vi "Sandbox.vi"() -> ()   [LabVIEW 2019, in "FPGA API.lvclass"]
uses:
  FPGA API.lvclass
  FPGA/TypeDef/DO index.ctl
  <vilib>/ptbypt/NI_PtbyPt.lvlib
panel:
  out "Ds":bool[](array[boolean])
  in  "#DO":T1 items=["DO 0 [KP1 [DO 0]]", "DO 1 [ON KP2 [DO 1]]", "DO 2 [ON KP3 [DO 2]]", "DO 3 [WATER Y18.1 [DO3]]", "DO 4 [WATER Y18.2 [DO4]]", "DO 5 [KP6 Y29.1 33.7]", "DO 6 [KP7 Y29.2 33.8]", "DO 7 [KP8 Y29.3 33.9]", "DO 8 [KP9 Y29.4  33.12]", "DO 9 [KP10 Y29.5 33.1]", "DO 10 [KP11 Y29.6 33.2]", "DO 11 [KP12 Y29.7  33.13]", "DO 12 [KP13 Y29.8  33.11]", "DO 13 [KP14 Y29.9 33.10]", "DO 14 [KP15 Y29.10  33.6]", "DO 15 [KP16 Y29.11  33.5]", "DO 16 [KP17 Y29.12  33.4]", "DO 17 [KP18 Y29.13 33.3]", "DO 18 [AIR KP19]", "DO 19 [STEP DRIVE EN KP20]", "DO 20 [KP21 Y44.1 OPEN]", "DO 21 [ KP22 Y44.1 CLOSE]", "DO 22 [ KP23 Y44.2 OPEN]", "DO 23", "DO 24 [STEP DRIVE 1]", "DO 25 [STEP DRIVE 2]"]
  out "Numeric":i32
  out "filter %":dbl
  out "avr %":dbl
  out "Raw %":dbl
  out "Waveform Chart":dbl[][](graph)
  out "DIs":bool[](array[boolean])
  out "dt(tiks) DI loop":u32
  out "dt(tiks) DO loop":u32
  out "dt(tiks) AI loop":u32
  out "error out":errorcluster
  in  "set":bool
  in  "Time uSec":u32
  in  "value":bool
  in  "stop":bool
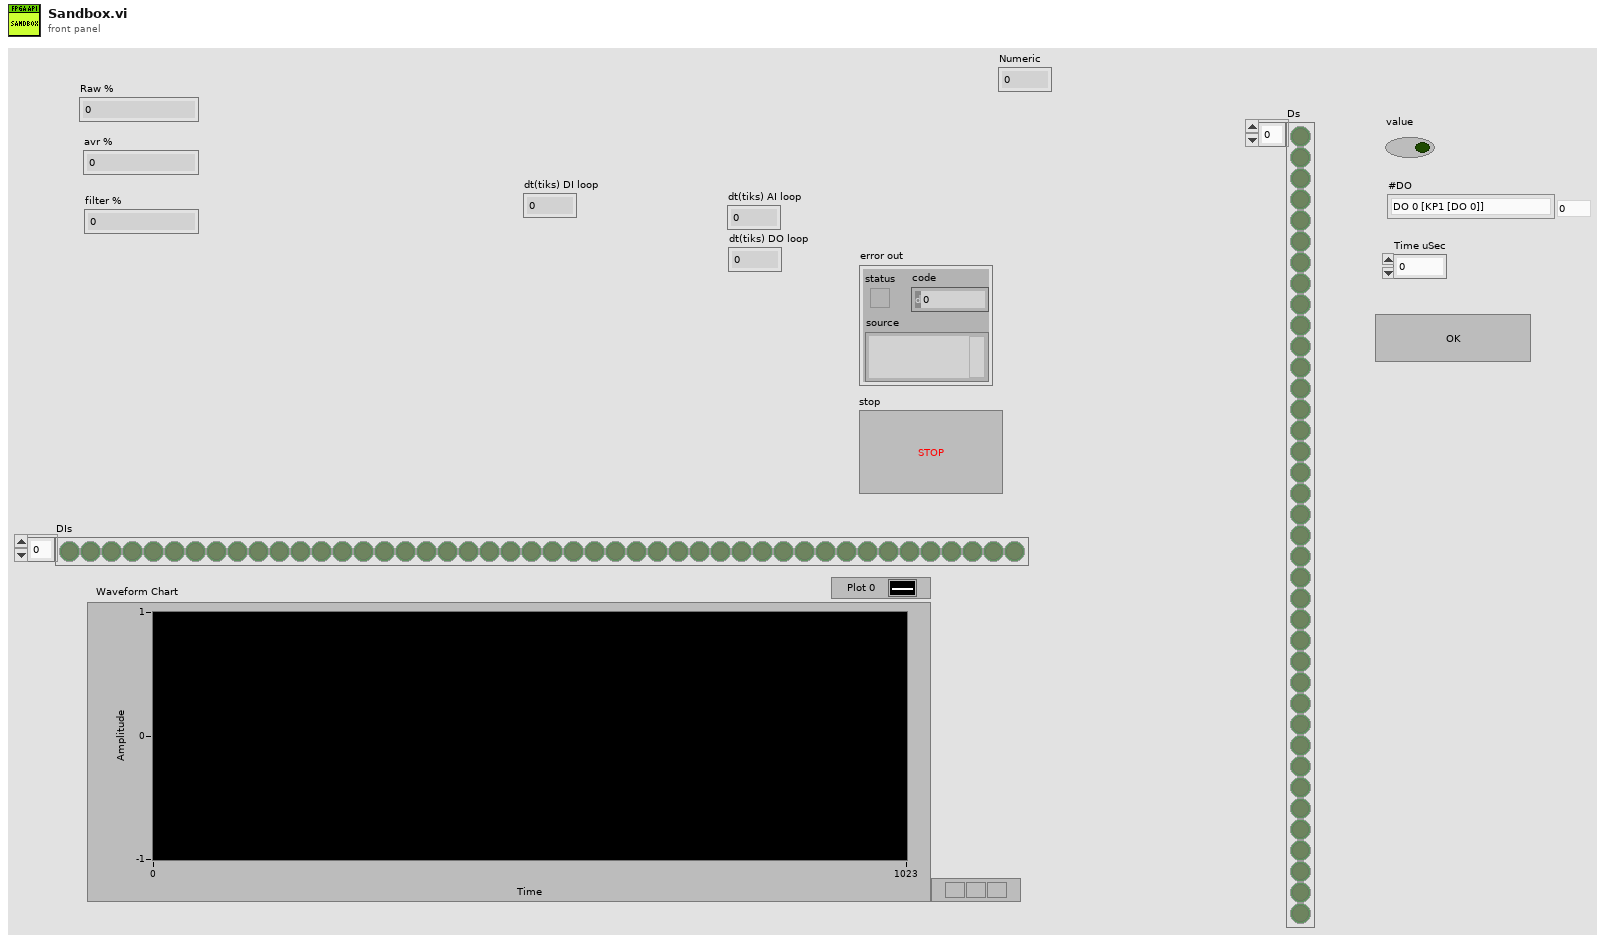
[diagram p1: front panel]
types:
  T1 = typedef "DO index.ctl" = u8
  T2 = cluster{"AI_0 L5.1":fxp<+/-,21,-4>, "AI_1 T4.1":fxp<+/-,21,-4>, "AI_2 L5.2":fxp<+/-,21,-4>, "AI_3 T4.2":fxp<+/-,21,-4>, "AI_4 V":fxp<+/-,21,-4>, "AI_5 P38.1":fxp<+/-,21,-4>, "AI_6 P38.2":fxp<+/-,21,-4>, "AI_7 P38.3":fxp<+/-,21,-4>, "AI_8 P41.1":fxp<+/-,21,-4>, "AI_9 P41.2":fxp<+/-,21,-4>, "AI_10 P41.3":fxp<+/-,21,-4>, "AI_11":fxp<+/-,21,-4>, "AI_12":fxp<+/-,21,-4>, "AI_13":fxp<+/-,21,-4>, "AI_14":fxp<+/-,21,-4>, "AI_15":fxp<+/-,21,-4>}
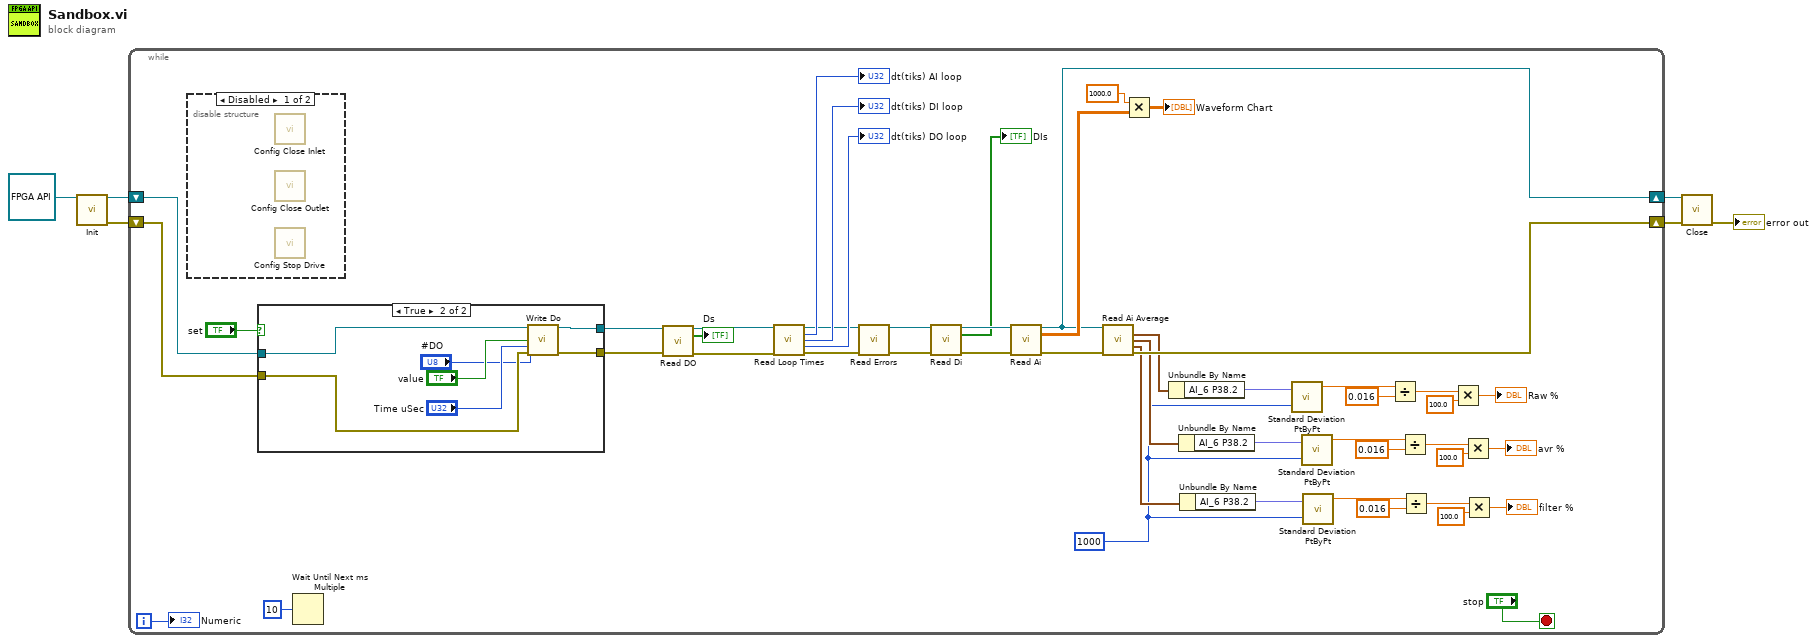
[diagram p0: block diagram]
diagram:
  n1 = call "Init.vi"("FPGA API in"=refnum<class "FPGA API.lvclass"> refnum) -> ("FPGA API out"=w5:refnum<class "FPGA API.lvclass">, "error out"=w4:errorcluster)  [unwired: 13 in]
  n2 = while {
    shift-right: [w38] -> w3
    shift-left: w5 -> [w42]
    shift-right: [w36] -> w2
    shift-left: w4 -> [w41]
    i -> [w13]
    stop <- "stop" stop-if-true
    w14 = 1000 ("sample length")
    n3 = disable-structure shown="Disabled" {
      frame Disabled {
        n4 = call "Config Close Inlet.vi"() -> ()  [unwired: 14 in, 2 out]
        n5 = call "Config Close Outlet.vi"() -> ()  [unwired: 14 in, 2 out]
        n6 = call "Config Stop Drive.vi"() -> ()  [unwired: 14 in, 2 out]
      }
      frame Enabled {
      }
    }
    n7 = case shown="True" "set" {
      tunnel: [w57 w64] -> w11
      tunnel: [w56 w63] -> w9
      tunnel: w42 -> [w57 w59]
      tunnel: w41 -> [w56 w62]
      frame False {
      }
      frame True {
        n8 = call "Write Do.vi"("FPGA API in"=w59, "#DO"="#DO", "value"="value", "Time uSec"="Time uSec", "error in (no error)"=w62) -> ("FPGA API out"=w64:refnum<class "FPGA API.lvclass">, "error out"=w63:errorcluster)  [unwired: 9 in]
      }
    }
    n9 = Wait Until Next ms Multiple(millisecond multiple=u32 10) -> ()  [unwired: 1 out]
    n10 = call "Read DO.vi"("FPGA API in"=w11, "error in (no error)"=w9) -> ("FPGA API out"=w10:refnum<class "FPGA API.lvclass">, "Ds"=→"Ds":bool[], "error out"=w8:errorcluster)  [unwired: 11 in]
    n11 = call "Read Loop Times.vi"("FPGA API in"=w10, "error in (no error)"=w8) -> ("FPGA API out"=w48:refnum<class "FPGA API.lvclass">, "dt(tiks) AI loop"=→"dt(tiks) AI loop":u32, "dt(tiks) DI loop"=→"dt(tiks) DI loop":u32, "dt(tiks) DO loop"=→"dt(tiks) DO loop":u32, "error out"=w49:errorcluster)  [unwired: 8 in, 1 out]
    n12 = call "Read Errors.vi"("FPGA API in"=w48, "error in (no error)"=w49) -> ("FPGA API out"=w47:refnum<class "FPGA API.lvclass">, "error out"=w46:errorcluster)  [unwired: 8 in, 4 out]
    n13 = call "Read Di.vi"("FPGA API in"=w47, "error in (no error)"=w46) -> ("FPGA API out"=w44:refnum<class "FPGA API.lvclass">, "DIs"=→"DIs":bool[], "error out"=w45:errorcluster)  [unwired: 11 in]
    n14 = call "Read Ai.vi"("FPGA API in"=w44, "error in (no error)"=w45) -> ("FPGA API out"=w38:refnum<class "FPGA API.lvclass">, "AI Data"=w40:dbl[][], "error out"=w37:errorcluster)  [unwired: 10 in, 1 out]
    n15 = call "Read Ai Average.vi"("FPGA API in"=w38, "error in (no error)"=w37) -> ("Raw"=w35:T2, "Average 1ms"=w16:T2, "Discrete Control Filter"=w15:T2, "error out"=w36:errorcluster)  [unwired: 9 in, 1 out]
    n16 = Multiply(x=1000.0, y=w40) -> (x*y=→"Waveform Chart":dbl[][])
    n17 = Unbundle By Name(w35) -> ("AI_6 P38.2"=w34:fxp<+/-,21,-4>)
    n18 = Unbundle By Name(w16) -> ("AI_6 P38.2"=w23:fxp<+/-,21,-4>)
    n19 = Unbundle By Name(w15) -> ("AI_6 P38.2"=w22:fxp<+/-,21,-4>)
    n20 = call <vilib>:"Standard Deviation PtByPt.vi"("x"=w34, "sample length"=w14) -> ("standard deviation"=w33:dbl)  [unwired: 1 in, 2 out]
    n21 = call <vilib>:"Standard Deviation PtByPt.vi"("x"=w23, "sample length"=w14) -> ("standard deviation"=w24:dbl)  [unwired: 1 in, 2 out]
    n22 = call <vilib>:"Standard Deviation PtByPt.vi"("x"=w22, "sample length"=w14) -> ("standard deviation"=w21:dbl)  [unwired: 1 in, 2 out]
    n23 = Divide(x=w33, y=0.016) -> (x/y=w31:dbl)
    n24 = Divide(x=w24, y=0.016) -> (x/y=w26:dbl)
    n25 = Divide(x=w21, y=0.016) -> (x/y=w19:dbl)
    n26 = Multiply(x=w31, y=100.0) -> (x*y=→"Raw %":dbl)
    n27 = Multiply(x=w26, y=100.0) -> (x*y=→"avr %":dbl)
    n28 = Multiply(x=w19, y=100.0) -> (x*y=→"filter %":dbl)
    "Numeric" <- w13
  }
  n29 = call "Close.vi"("FPGA API in"=w3, "error in (no error)"=w2) -> ("error out"=→"error out":errorcluster)  [unwired: 12 in, 1 out]
